vi "Out_S2F41.vi"(8 "error in (no error)":errorcluster, 10 "S2F41":T1, 11 "S2 Message Class in":refnum<class "S2 Message Class.lvclass">) -> (0 "error out":errorcluster, 3 "S2 Message Class out":refnum<class "S2 Message Class.lvclass">)   [LabVIEW 2020, in "SECS Communication.lvlib" / "S2 Message Class.lvclass"]
uses:
  S2 Message Class.lvclass
  D:/Dropbox/SECS/SECS_GEM v1.0.6/Com/SECS Communication/SECS-II Class/SECS-II Class.lvclass
  S2F41.ctl
  SECS-II Class/Data Message_List.vi
  SECS-II Class/Data Message_ASCII.vi
  SECS-II Class/SECS-II Class.lvclass
  D:/Dropbox/SECS/SECS_GEM v1.0.6/Com/SECS Communication/S2 Message Class/S2 Message Class.lvclass
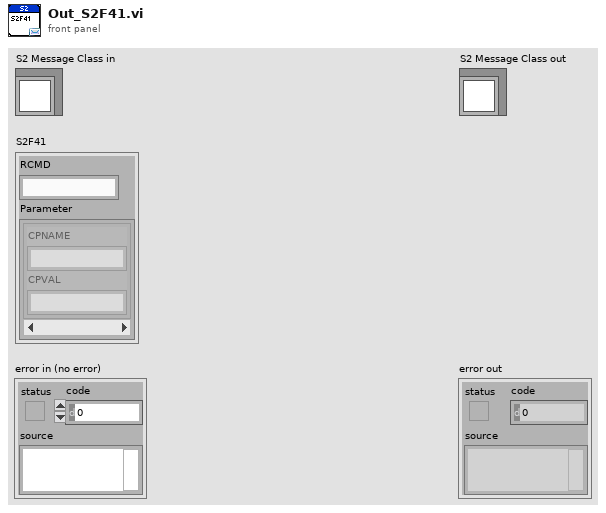
[diagram p1: front panel]
types:
  T1 = typedef "SECS Communication.lvlib/S2 Message Class.lvclass/S2F41.ctl" = cluster{"RCMD":string, "Parameter":cluster{"CPNAME":string, "CPVAL":string}[]}
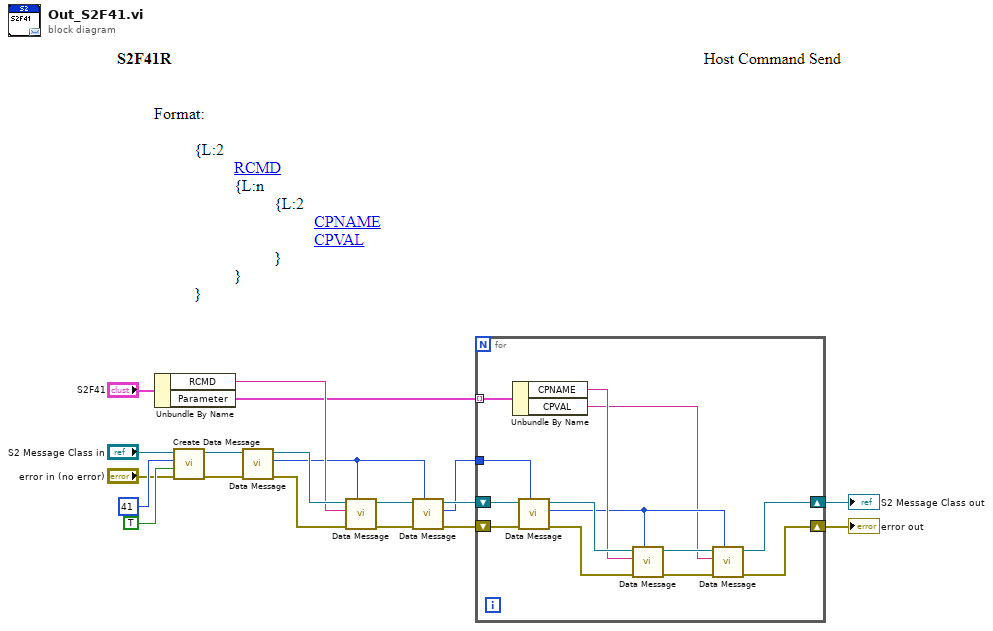
[diagram p0: block diagram]
diagram:
  n1 = Unbundle By Name("S2F41") -> ("RCMD"=w10:string, "Parameter"=w3:cluster{"CPNAME":string, "CPVAL":string}[])
  n2 = call "Create Data Message.vi"("error in (no error)"="error in (no error)", "W-Bit"=TRUE, "Function"=u8 41, "SECS-II Class in"="S2 Message Class in") -> ("error out"=w14:errorcluster, "SECS-II Class out"=w17:refnum<class "S2 Message Class.lvclass">)  [unwired: 6 in]
  n3 = call-poly "Data Message.vi"("error in"=w14, "SECS-II Class in"=w17) -> ("error out"=w11:errorcluster, "Index"=w7:i32, "SECS-II Class out"=w12:refnum<class "S2 Message Class.lvclass">)  [unwired: 7 in]
  n4 = call-poly "Data Message.vi"("Parent Index"=w7, "error in"=w11, "Data"=w10, "SECS-II Class in"=w12) -> ("error out"=w8:errorcluster, "SECS-II Class out"=w9:refnum<class "S2 Message Class.lvclass">)  [unwired: 6 in]
  n5 = call-poly "Data Message.vi"("Parent Index"=w7, "error in"=w8, "SECS-II Class in"=w9) -> ("error out"=w5:errorcluster, "Index"=w4:i32, "SECS-II Class out"=w6:refnum<class "S2 Message Class.lvclass">)  [unwired: 6 in]
  n6 = for {
    shift-right: [w20] -> w1
    shift-left: w5 -> [w32]
    shift-right: [w21] -> w2
    shift-left: w6 -> [w31]
    tunnel: w4 -> [w30]
    tunnel: w3 -> [w27] mode=indexing
    n7 = Unbundle By Name(w27) -> ("CPNAME"=w26:string, "CPVAL"=w22:string)
    n8 = call-poly "Data Message.vi"("Parent Index"=w30, "error in"=w32, "SECS-II Class in"=w31) -> ("error out"=w29:errorcluster, "Index"=w23:i32, "SECS-II Class out"=w28:refnum<class "S2 Message Class.lvclass">)  [unwired: 6 in]
    n9 = call-poly "Data Message.vi"("Parent Index"=w23, "error in"=w29, "Data"=w26, "SECS-II Class in"=w28) -> ("error out"=w24:errorcluster, "SECS-II Class out"=w25:refnum<class "S2 Message Class.lvclass">)  [unwired: 6 in]
    n10 = call-poly "Data Message.vi"("Parent Index"=w23, "error in"=w24, "Data"=w22, "SECS-II Class in"=w25) -> ("error out"=w20:errorcluster, "SECS-II Class out"=w21:refnum<class "S2 Message Class.lvclass">)  [unwired: 6 in]
  }
  "error out" <- w1
  "S2 Message Class out" <- w2
